vi "FindInstrConnect.vi"(4 "Column #":i8, 5 "ArrayBoolian":bool[][](array[boolean])) -> (0 "Numeric":i64, 1 "String":string, 2 "Path":path)   [LabVIEW 2017]
uses:
  <vilib>/Utility/file.llb/Read From Spreadsheet File (I64).vi
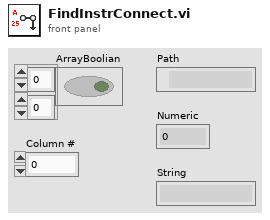
[diagram p1: front panel]
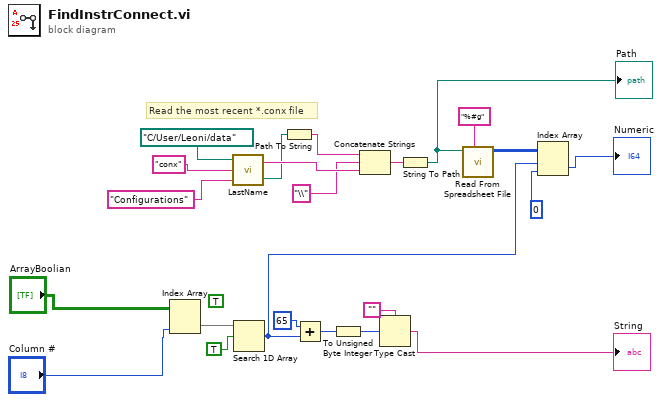
[diagram p0: block diagram]
diagram:
  (unwired) TRUE
  # "Read the most recent *.conx file"
  n1 = Index Array(array="ArrayBoolian", index (col)="Column #") -> (element=w1:bool[])  [unwired: 1 in]
  n2 = call "LastName.vi"("Custom Folder"="Configurations", "Extention"="conx", "User Data Folder"=path "C:/User/Leoni/data") -> ("created path"=w14:path, "String"=w15:string)
  n3 = Search 1D Array(1D array=w1, element=TRUE) -> (index of element=w21:i32)  [unwired: 1 in]
  n4 = Path To String(path=w14) -> (string=w10:string)
  n5 = Add(x=65, y=w21) -> (x+y=w5:i32)
  n6 = To Unsigned Byte Integer(number=w5) -> (unsigned 8bit integer=w6:u8)
  n7 = Concatenate Strings(w10, "\\", w15) -> (w12:string)
  n8 = Type Cast(type="", x=w6) -> (*(type *) &x=→"String":string)
  n9 = String To Path(string=w12) -> (path=w19:path)
  "Path" <- w19
  n10 = call-poly <vilib>:"Read From Spreadsheet File.vi"("format (%d)"="%#g", "file path (dialog if empty)"=w19) -> ("all rows"=w20:i64[][])  [unwired: 5 in, 4 out]
  n11 = Index Array(array=w20, index (row)=w21, index (col)=0) -> (element=→"Numeric":i64)
